vi "PH_PILS.set color of beamline.vi"(0 "i ref in":refnum<vi>, 5 "error in":errorcluster) -> (14 "i ref out":refnum<vi>, 19 "error out":errorcluster)   [LabVIEW 2014, in "PH_PILS.lvlib"]
doc: "This VI sets the cvolor of beamline elements."
uses:
  PH_PILS.lvlib
  PH_Common/PH_Common.lvlib
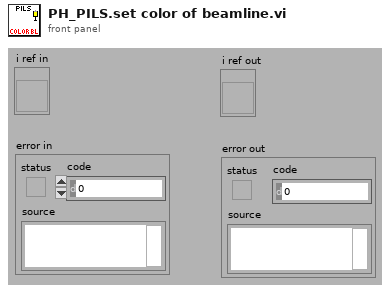
[diagram p1: front panel]
types:
  T1 = typedef "PH_PILS.lvlib/PH_PILS.i attribute.ctl" = cluster{"Boolean":cluster{"GUI Ref":refnum<vi>, "Status":i32}[], "GUI Refs Exp. Shutters":cluster{"1":refnum<vi>, "2":refnum<vi>, "3":refnum<vi>, "4":refnum<vi>}, "Tristate2Run GUI Refs":refnum<vi>[], "EO-Likes":cluster{"GUI Ref":refnum<vi>, "Status":i32}[], "Operation Mode":cluster{"Operation Mode":T2, "GUI":cluster{"Ref State":refnum<vi>, "Ref":refnum<vi>}, "Servicemode":cluster{"Tagname":string, "Status":i32}, "Labormode":cluster{"Tagname":string, "Status":i32}, "Searchmode":cluster{"Tagname":string, "Status":i32}, "Shotmode":cluster{"Tagname":string, "Status":i32}}, "Submode":cluster{"Submode":T3, "GUI":cluster{"Ref State":refnum<vi>, "Ref":refnum<vi>}, "Submode":cluster{"Tagname":string, "Status":i32}}, "Experiment":cluster{"Experiment":enum16{"unknown", "intern", "4 (Z6)", "3", "2", "1"}, "GUI":cluster{"Ref State":refnum<vi>, "Ref":refnum<vi>}, "intern":cluster{"Tagname":string, "Status":i32}, "Exp 4":cluster{"Tagname":string, "Status":i32}, "Exp 3":cluster{"Tagname":string, "Status":i32}, "Exp 2":cluster{"Tagname":string, "Status":i32}, "Exp 1":cluster{"Tagname":string, "Status":i32}}, "TristateNormal":cluster{"GUI Ref":refnum<vi>, "Status":i32}[], "Door Tags":cluster{"GUI Ref":refnum<vi>, "Status":i32}[], "GUIlessTags":cluster{"Name":string, "Status":i32}[], "Beamline GUI Refs":refnum<vi>[], "Special Boolean":cluster{"GUI Ref":refnum<vi>, "Status":i32}[], "Laserpower":cluster{"GUI Ref":refnum<vi>, "Status":i32}[], "Shutter":cluster{"GUI Ref":refnum<vi>, "Status":i32}[], "Tristate EO Like":cluster{"GUI Ref":refnum<vi>, "Status":i32}[], "PP":cluster{"GUI Ref":refnum<vi>, "Status":i32, "Head Ref":refnum<vi>, "Slider Ref":refnum<vi>}[], "Switch Knobs":cluster{"GUI Ref":refnum<vi>, "Status":i32}[], "Latch Knob GUI Refs":refnum<vi>[], "FailureCounter":i32, "Enabled Status":cluster{"Laser":i32, "PreAmp":i32, "MainAmp":i32}, "Mercury":refnum<vi>, "Instance Rods":string, "Logfile":path, "Beckhoff-Instance Internal":string, "Beckhoff-Instance External":string, "Enabling Rights":cluster{"Name":string, "Password":string, "PA?":bool, "MA?":bool, "Exp?":bool}[]}
  T2 = typedef "PH_PILS.lvlib/PH_PILS.Operation Mode.ctl" = enum16{"unknown", "Service", "Labor", "Search", "Shot"}
  T3 = typedef "PH_PILS.lvlib/PH_PILS.Submode.ctl" = enum16{"unknown", "HV-Normal", "HV-Test"}
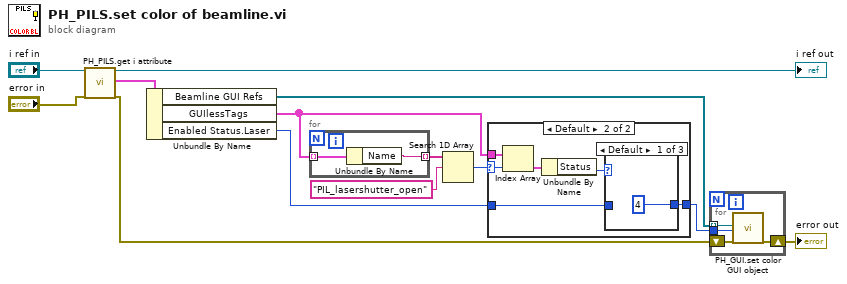
[diagram p0: block diagram]
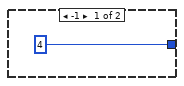
[diagram p2: hidden frame]
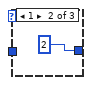
[diagram p3: hidden frame]
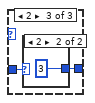
[diagram p4: hidden frame]
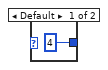
[diagram p5: hidden frame]
diagram:
  n1 = call "PH_PILS.get i attribute.vi"("i ref in"="i ref in", "error in (no error)"="error in") -> ("i ref out"=→"i ref out":refnum<vi>, "i attribute"=w9:T1, "error out"=w11:errorcluster)  [unwired: 15 in]
  n2 = Unbundle By Name(w9) -> ("Beamline GUI Refs"=w7:refnum<vi>[], "GUIlessTags"=w6:cluster{"Name":string, "Status":i32}[], "Enabled Status.Laser"=w2:i32)
  n3 = for {
    tunnel: w6 -> [w15] mode=indexing
    tunnel: [w14] -> w5 mode=indexing
    n4 = Unbundle By Name(w15) -> ("Name"=w14:string)
  }
  n5 = Search 1D Array(1D array=w5, element="PIL_lasershutter_open") -> (index of element=w1:i32)  [unwired: 1 in]
  n6 = case shown="Default" w1 {
    selector: w1 -> [_ w17]
    tunnel: w6 -> [_ w22]
    tunnel: [4 ("Status") w19] -> w3
    tunnel: w2 -> [_ w18]
    frame -1 {
    }
    frame Default {
      n7 = Index Array(array=w22, index=w17) -> (element=w21:cluster{"Name":string, "Status":i32})
      n8 = Unbundle By Name(w21) -> ("Status"=w20:i32)
      n9 = case shown="Default" w20 {
        tunnel: [4 ("Status") 2 ("Status") w25] -> w19
        tunnel: w18 -> [_ _ w26]
        frame Default {
        }
        frame 1 {
        }
        frame 2 {
          n10 = case shown="2" w26 {
            tunnel: [4 ("Status") 3 ("Status")] -> w25
            frame Default {
            }
            frame 2 {
            }
          }
        }
      }
    }
  }
  n11 = for {
    tunnel: w7 -> [w30] mode=indexing
    shift-right: [w31] -> w8
    shift-left: w11 -> [w32]
    tunnel: w3 -> [w29]
    n12 = call "PH_GUI.set color GUI object.vi"("GUI object Ref"=w30, "State"=w29, "error in (no error)"=w32) -> ("error out"=w31:errorcluster)  [unwired: 16 in]
  }
  "error out" <- w8
